vi "G heatmap=f(orbital angle, E_mol)_on Bi.vi"() -> ()   [LabVIEW 2016]
uses:
  <vilib>/Math Plots/3D Math Plots/3D Contour/3D Contour XCtrl/3D Contour.xctl
  <vilib>/Math Plots/3D Math Plots/3D Contour/3D Contour Datatype/3D Contour Datatype.lvclass
  <vilib>/Analysis/1siggen.llb/Ramp Pattern by Samples.vi
  <vilib>/Math Plots/3D Math Plots/3D Contour/3D Contour Datatype/Public/Plot Helper (Vector).vi
  <vilib>/Utility/file.llb/Write Delimited Spreadsheet (DBL).vi
  <vilib>/Analysis/NI_AALBase.lvlib
  <vilib>/Math Plots/3D Math Plots/3D Plot/3D Plot Datatype/3D Plot Datatype.lvclass
  <vilib>/Analysis/NI_AALPro.lvlib
panel:
  out "Array 3":dbl[](array[numeric])
  out "Array 2":dbl[](array[numeric])
  in  "turn on dyz":bool
  in  "turn on dz2":bool=TRUE
  out "<= min[dnn]?":bool
  out "e_FMO after dz2\n(vs. E_F) <=>\nintercept on E\ndz2 band-mol":dbl
  out "e_FMO after sp \n(vs. E_F) <=>\nintercept on E\nsp band-mol":dbl
  out "intercept on E\ndyz band-mol":dbl
  out "graphical sol_dyz band-mol":cluster{"Ramp Pattern":dbl[], dbl[]}[](graph)
  out "delta shift by d band \n(w.r.t. e_FMO coupled to s/p then dz2 )":dbl
  out "unweighted dyz SDOS \n@intercept":dbl
  in  "e_dyz band \n(vs. E_F)":dbl=-3.41 format="%.2f"
  in  "t_dyz band":dbl=1.1 format="%.2f"
  out "dyz SDOS top \n(/eV/atom)":dbl=0.793 format="%.3f"
  out "log(G/G0)=f(angle, e_iso) for t(sp-head)":refnum<class "3D Plot Datatype.lvclass">[](xcontrol)
  in  "min dnn (A)\nby induction":dbl=2.1 format="%.3g"
  out "Array":dbl[](array[numeric])
  out "peak value":dbl
  out "unweighted sp(xy) SDOS \n@ intercept":dbl
  out "t^2_sp(xy)-mol":dbl
  out "s/p(xy) SDOS top (/eV/atom)":dbl=0.118 format="%.3f"
  in  "e_s/p(xy) band (vs. E_F)":dbl=0.15 format="%.2f"
  in  "t_s/p(xy) band":dbl=2.99 format="%.2f"
  out "angle > ini?":bool
  in  "dnn shrinking \nrate\n(A/increment)":dbl=0.029 format="%.4g"
  in  "induction rate\n(_-fold of increment)":dbl=3.42 format="%.3g"
  in  "orbital angle \nstarting induction":dbl=47.14 format="%.2g"
  out "unweighted dz2 SDOS \n@intercept":dbl
  out "unweighted sp(z) SDOS \n@ intercept":dbl
  out "dz2 SDOS top \n(/eV/atom)":dbl=0.793 format="%.3f"
  out "s/p(z) SDOS top (/eV/atom)":dbl=0.118 format="%.3f"
  in  "eta scaling for sp":dbl=0.417 format="%.3f"
  in  "name (d band)":string="on Bi 6dz2"
  in  "saving path_heatmap (d band)":path=path "C:/Users/NTU/Desktop/project_BiUPD & PbUPD/modelling/general map on BiUPD"
  in  "save heatmap \n(d band)?":bool
  out "final ELA(angle, e_iso  for t(sp-head))":refnum<class "3D Plot Datatype.lvclass">[](xcontrol)
  out "delta(angle, e_iso) for t(d-head)_sum dz2 & dyz":refnum<class "3D Plot Datatype.lvclass">[](xcontrol)
  out "delta(angle, e_iso) for t(sp-head)_only pz":refnum<class "3D Plot Datatype.lvclass">[](xcontrol)
  out "delta shift by dz2 band \n(w.r.t. e_FMO coupled to s/p )":dbl
  out "delta shift by \nsp band":dbl
  in  "dnn (pi) dyz":dbl=100.0 format="%0.2f"
  out "Gamma(angle, e_iso) for t(sp-head)_sum pz & py":refnum<class "3D Plot Datatype.lvclass">[](xcontrol)
  out "e_FMO (vs. E_F)":dbl
  out "log(G/G0) matrix":dbl[][](array[numeric])
  in  "tilt (mol axis - Z axis)":dbl format="%0.2f"
  out "final ELA(angle, e_iso)  for t(d-head)":refnum<class "3D Plot Datatype.lvclass">[](xcontrol)
  out "Gamma(angle, e_iso) for t(d-head)_sum dz2 & dyz":refnum<class "3D Plot Datatype.lvclass">[](xcontrol)
  out "log(G/G0)=f(angle, e_iso) for t(d-head)":refnum<class "3D Plot Datatype.lvclass">[](xcontrol)
  out "e_FMO (y)":dbl[](array[numeric])
  out "angle\narray\nfor sigma":dbl[](array[numeric])
  in  "create heatmap":bool=TRUE
  in  "name (sp band)":string="on Bi 6pz 6pxy"
  in  "save heatmap \n(sp band)?":bool
  in  "saving path_heatmap (sp band)":path=path "C:/Users/NTU/Desktop/project_BiUPD & PbUPD/modelling/general map on BiUPD"
  in  "lower angle":dbl=-90.0 format="%_3g"
  in  "upper angle":dbl=90.0 format="%_3g"
  in  "angle increment":dbl=0.5 format="%_3g"
  in  "lower e_iso FMO":dbl=-3.0 format="%_3g"
  in  "upper e_iso FMO":dbl=3.0 format="%_3g"
  in  "increment_iso FMO":dbl=0.03 format="%_3g"
  out "t^2_dz2-mol":dbl
  out "FWHM (eV)":dbl
  in  "dnn (pi) p(xy)":dbl=2.61 format="%0.2f"
  in  "WF (eV) vs. Fermi":dbl format="%.2f"
  out "t^2_sp(z)-mol":dbl
  out "t_s/p(xy)-mol":dbl
  in  "eta (pi)":i32=3
  in  "start (eV)":dbl=-20.0 format="%.2f"
  in  "dnn (sigma) sp(z)":dbl=2.61 format="%0.2f"
  in  "eta (sigma)":i32=2
  out "t_sp(z)-mol":dbl
  out "intercept on E\nsp band-mol":dbl
  out "graphical sol_sp band-mol":cluster{"Ramp Pattern":dbl[], dbl[]}[](graph)
  in  "e_s/p(z) band (vs. E_F)":dbl=-0.6 format="%.2f"
  in  "t_s/p(z) band":dbl=2.71 format="%.2f"
  out "E":dbl[](array[numeric])
  out "t^2_dyz-mol":dbl
  out "final ELA (eV), via \n(1) sp intercept\n(2) dz2 intercept\n(3) dyz intercept":dbl
  in  "ELD AO (pi w/ FMO) - Z axis":dbl format="%0.2f"
  out "graphical sol_dz2 band-mol":cluster{"Ramp Pattern":dbl[], dbl[]}[](graph)
  out "intercept on E\ndz2 band-mol":dbl
  out "t_dz2-mol":dbl
  out "t_dyz-mol":dbl
  in  "e_dz2 band \n(vs. E_F)":dbl=14.41 format="%.2f"
  in  "t_dz2 band":dbl=5.1 format="%.2f"
  in  "eta (pi)":i32=2
  in  "ELD AO (sigma w/ FMO) - Z axis":dbl format="%0.2f"
  in  "mol backbone (# n)":dbl=8.0 format="%.2f"
  in  "beta (per n)":dbl=1.0 format="%.2f"
  out "conductance G0 \n(on E_F, low bias)":dbl format="%#.3e"
  in  "eta (sigma)":i32=1
  out "transmission T(E)":cluster{"Ramp Pattern":dbl[], dbl[]}(graph)
  in  "d state R (Ang)":dbl=1.0099999999999998 format="%0.2f"
  in  "FMO - mol axis":dbl format="%0.2f"
  in  "dnn (sigma) dz2":dbl=2.61 format="%0.2f"
  in  "samples":i32=10000
  in  "end (eV)":dbl=20.0 format="%_3g"
  # "for eld-head hopping integral: \nHarrsion and S-K"
  # "for ELA & Gamma: Hilbert & Newns-Anderson-Grimley graphical method"
  # "for T(E) and G(E_F)\nLandauer formula"
  # "logG heatmap = f(t(number basis), e_iso FMO)"
  # "step2. dz2 band-mol \ncoupling"
  # "step3. dyz band-mol coupling"
  # "step1. s/p band-mol coupling"
  # "Harrison LCAO hopping integral (V)"
  # "exp decay for backbone"
  # "internuclear \nspacing, dnn (Ang)"
  # "off-diagonal\nelement type"
  # "FMO-s/p eld AO"
  # "1 sp_sigma\n2 pp_sigma"
  # "1 sp_pi =0\n2 pp_sigma\n3 pp_pi"
  # "FMO-d eld AO"
  # "1 pd_sigma\n2 pd_pi"
  # "BiUPD dz2\nc: 14.41\nt: 5.10"
  # "the avg of the two \nshould be e_ELD (vs. E_F)"
  # "BiUPD dz2\nc: 14.41\nt: 5.10"
  # "Au dyz\nc: -3.41\nt: 1.10"
  # "Au s\nc: -0.04\nt: 5.03"
  # "Au py\nc: 11.01\nt: 6.11"
  # "BiUPD pz\nc: -0.60\nt: 2.71"
  # "BiUPD py\nc: 0.15\nt: 2.99"
  # "1 pd_sigma\n2 pd_pi"
  # "to switch off certain interactions => set very large d (Ang)"
  # "for heatmap"
  # "for inducting effect"
  # "e_iso FMO\n (vs. E_F)"
  # "angle basis"
  # "induction"
  # "dnn"
  # "note: this is\nnot simply \nthe Gamma"
  # "to switch off certain effects => set 1 or 0"
  # "Slater-Koster t =f(bond angle)"
  # "+"
  # "一"
  # "FMO - ELD AO \nangle (sigma)"
  # "="
  # "FMO - ELD AO\n angle (pi)"
  # "="
  # "inverse \ncolor scale"
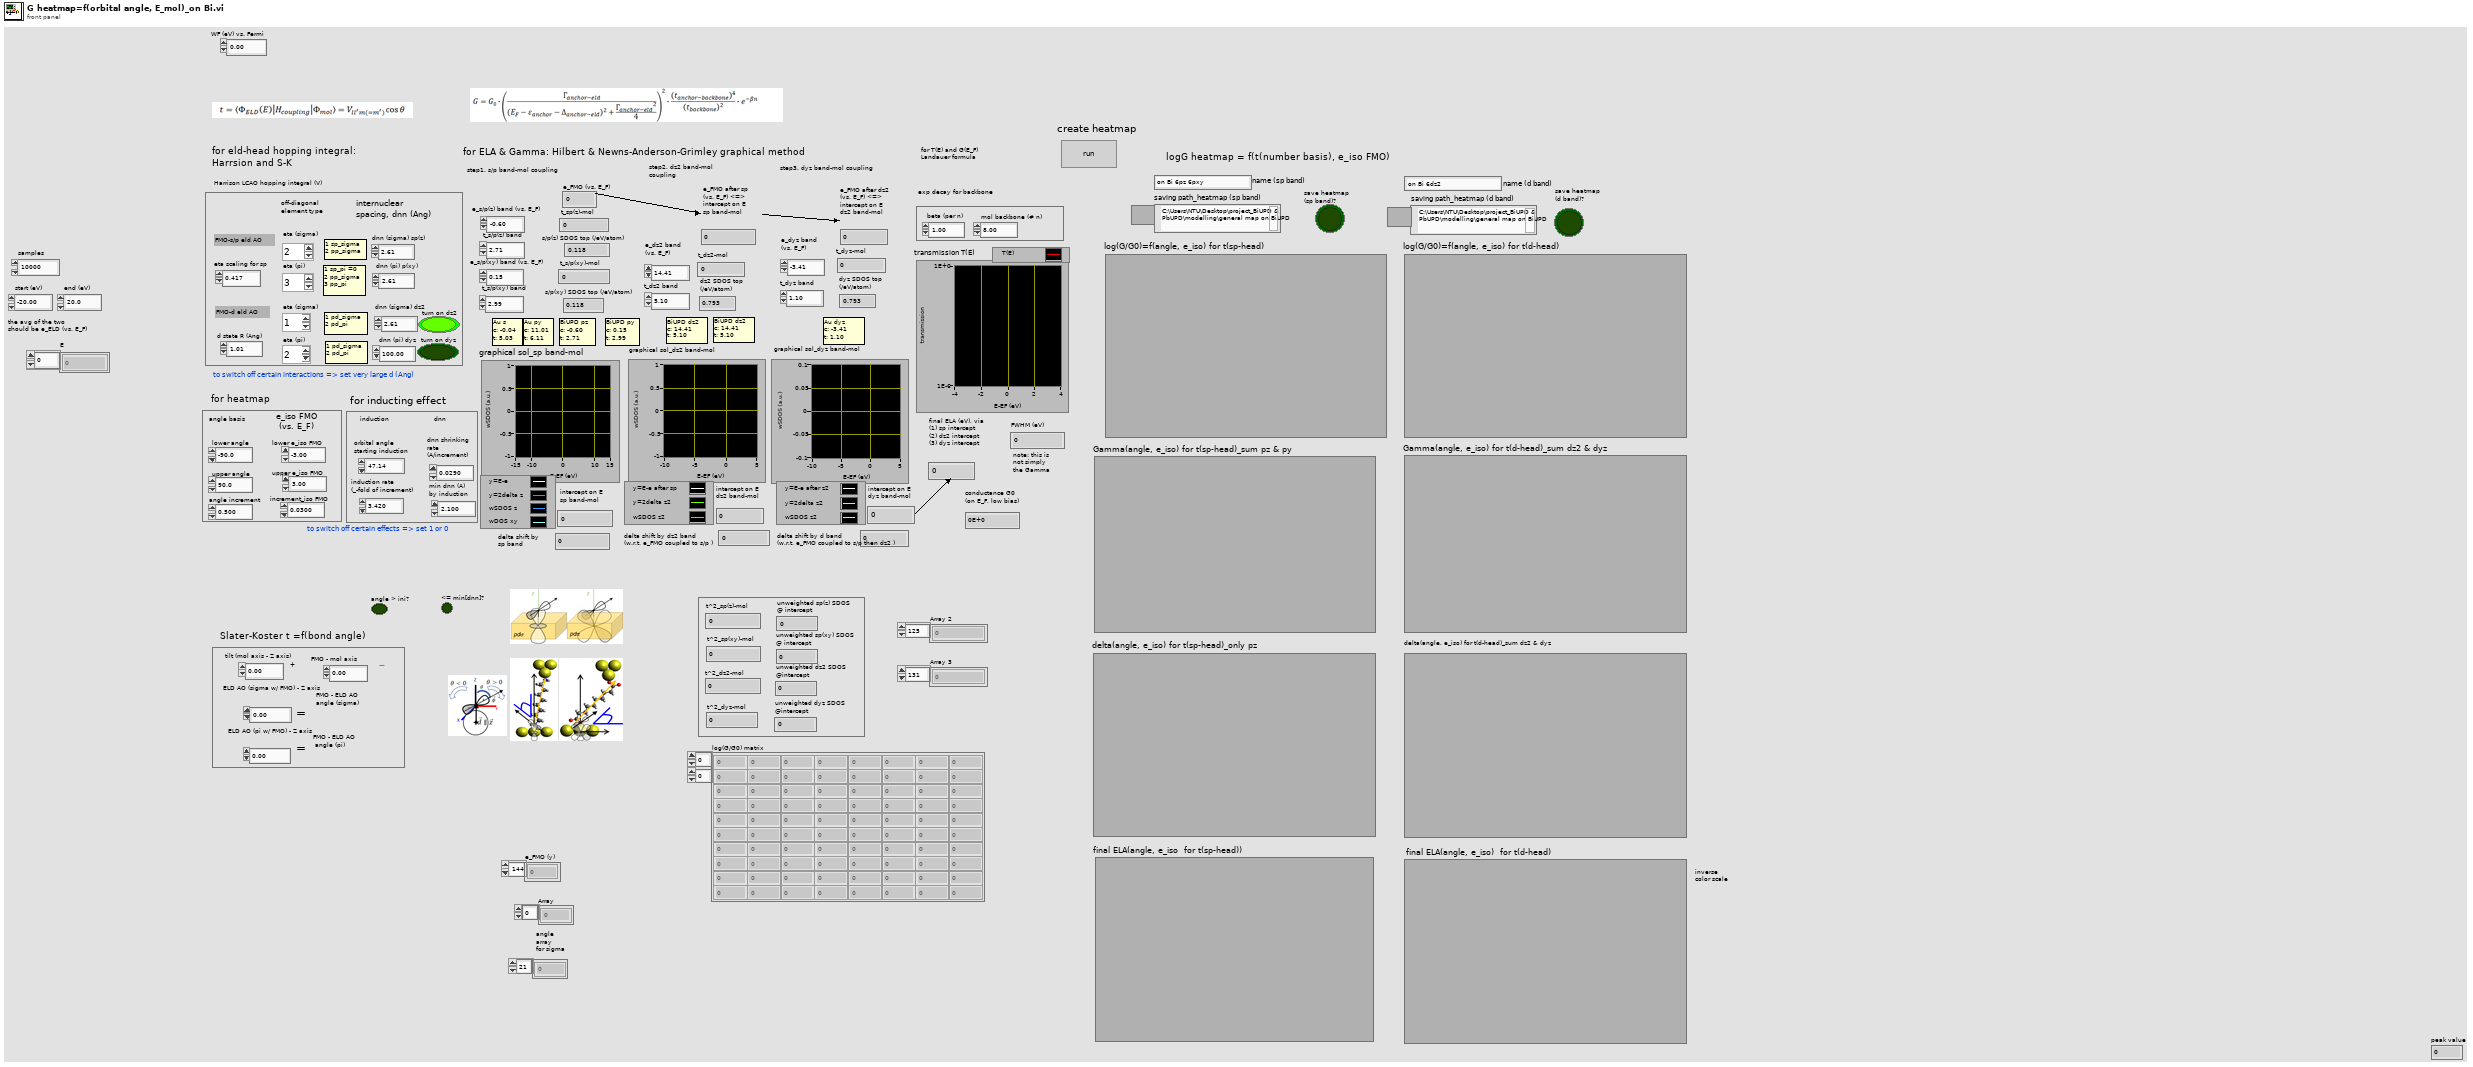
[diagram p1: front panel]
types:
  T1 = cluster{"Ramp Pattern":dbl[], "Hilbert{X}":dbl[]}
  T2 = cluster{"Ramp Pattern":dbl[], "Hilbert{X}":dbl[]}[]
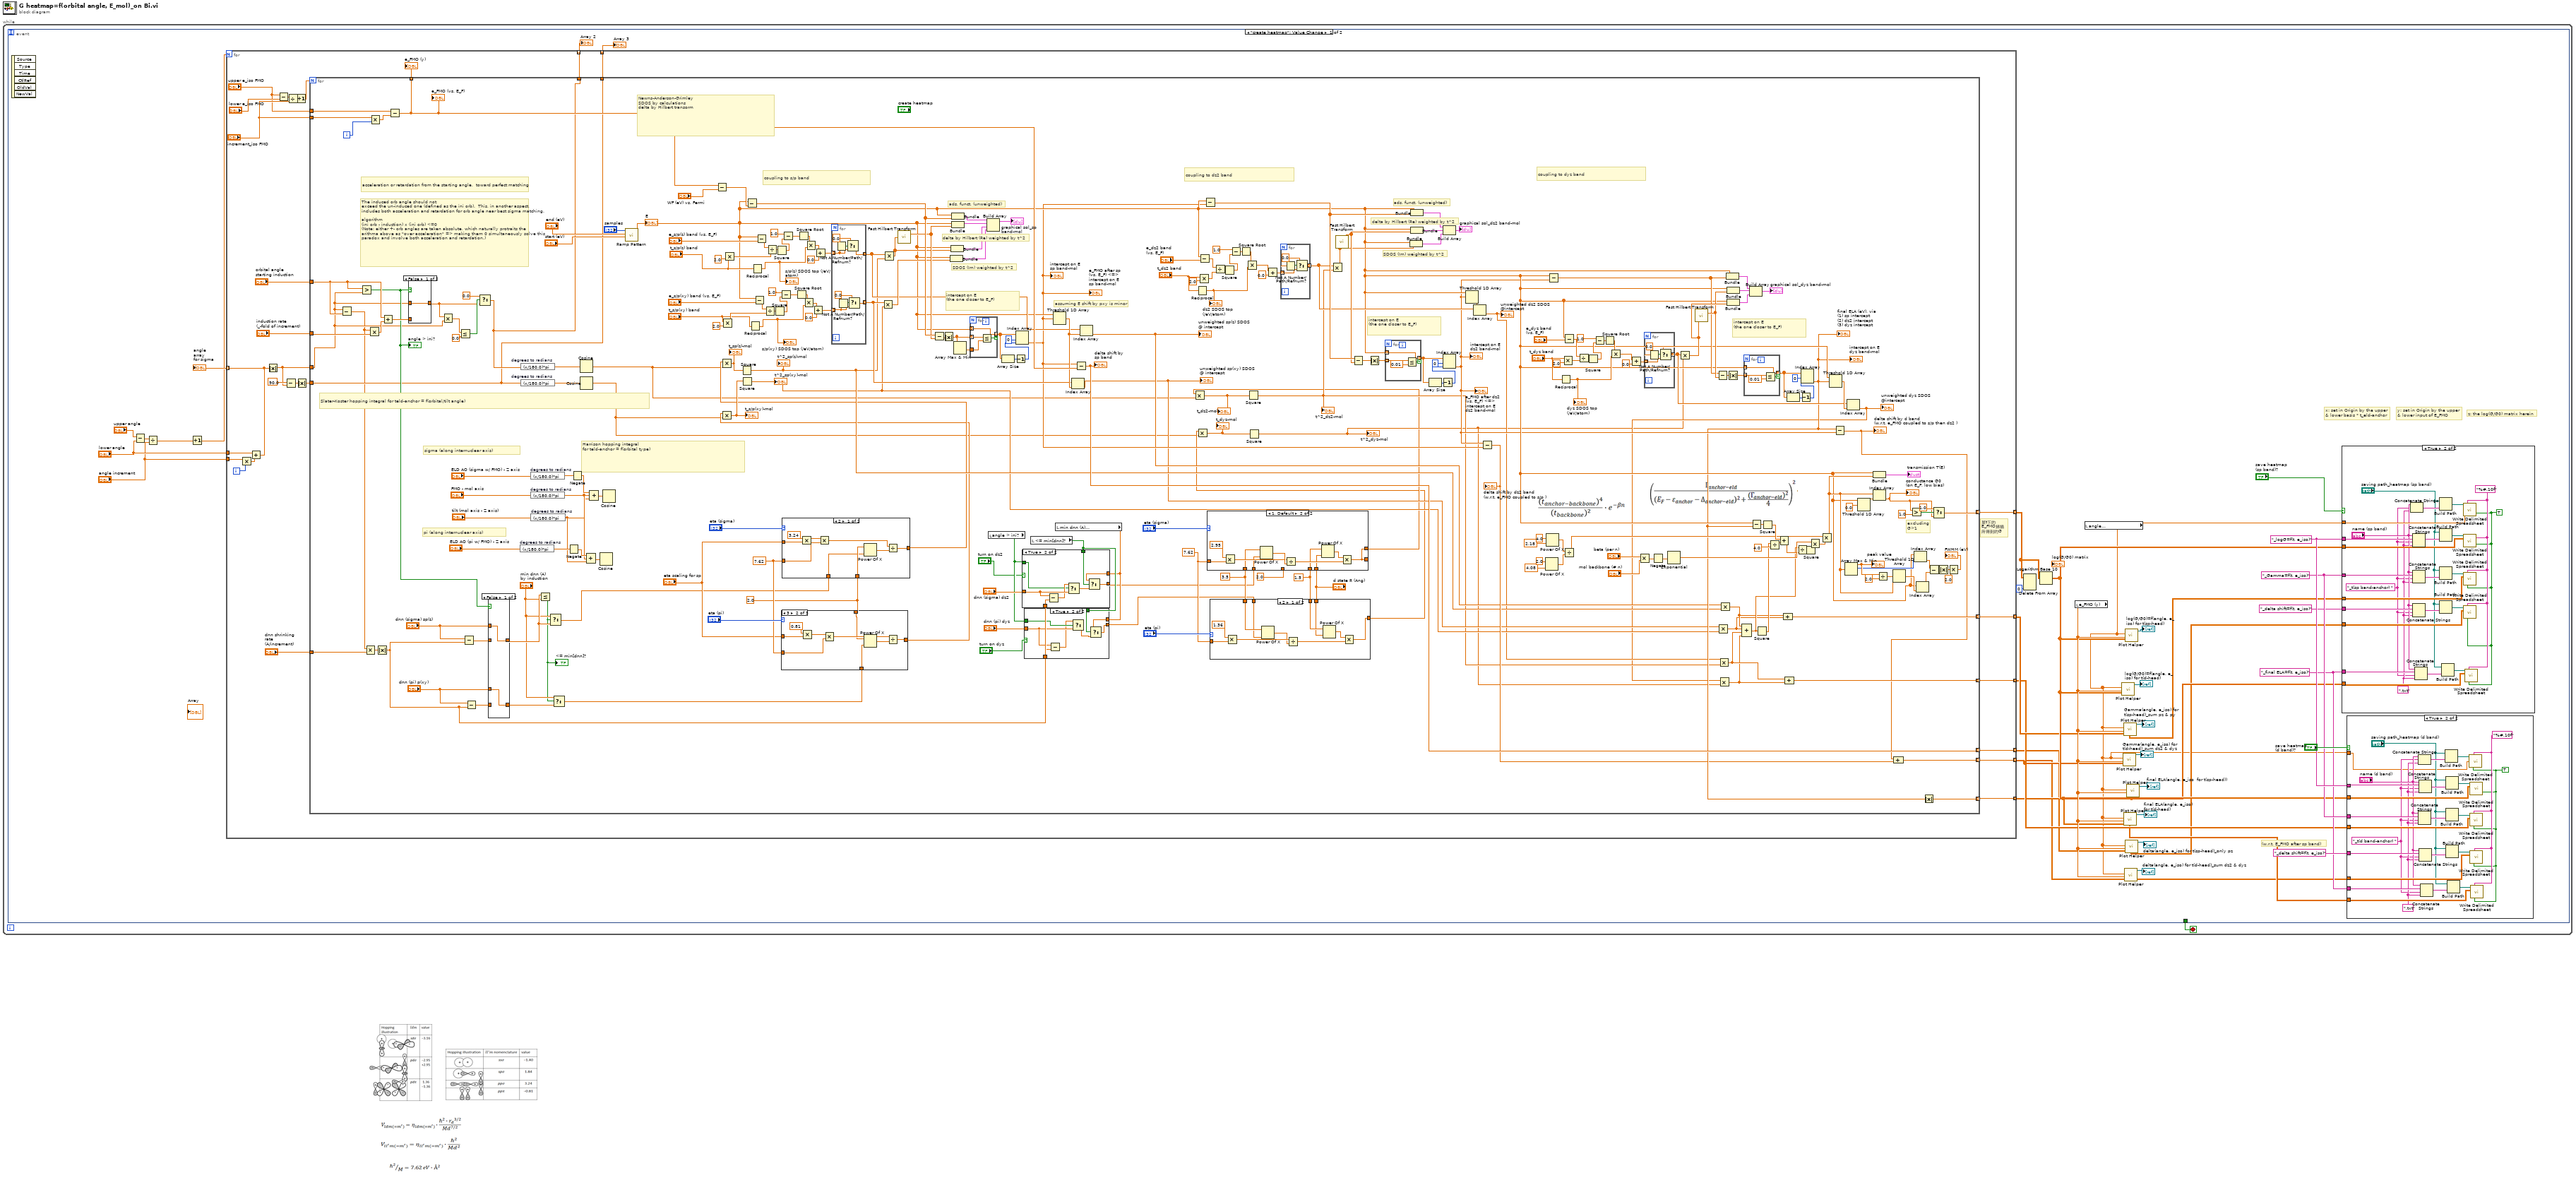
[diagram p0: block diagram]
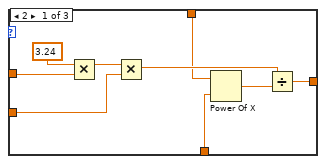
[diagram p8: hidden frame]
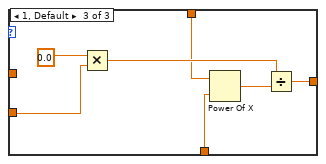
[diagram p9: hidden frame]
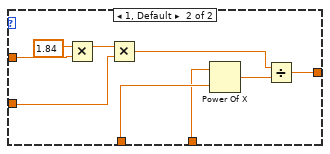
[diagram p10: hidden frame]
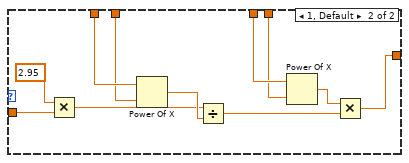
[diagram p11: hidden frame]
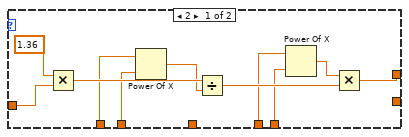
[diagram p12: hidden frame]
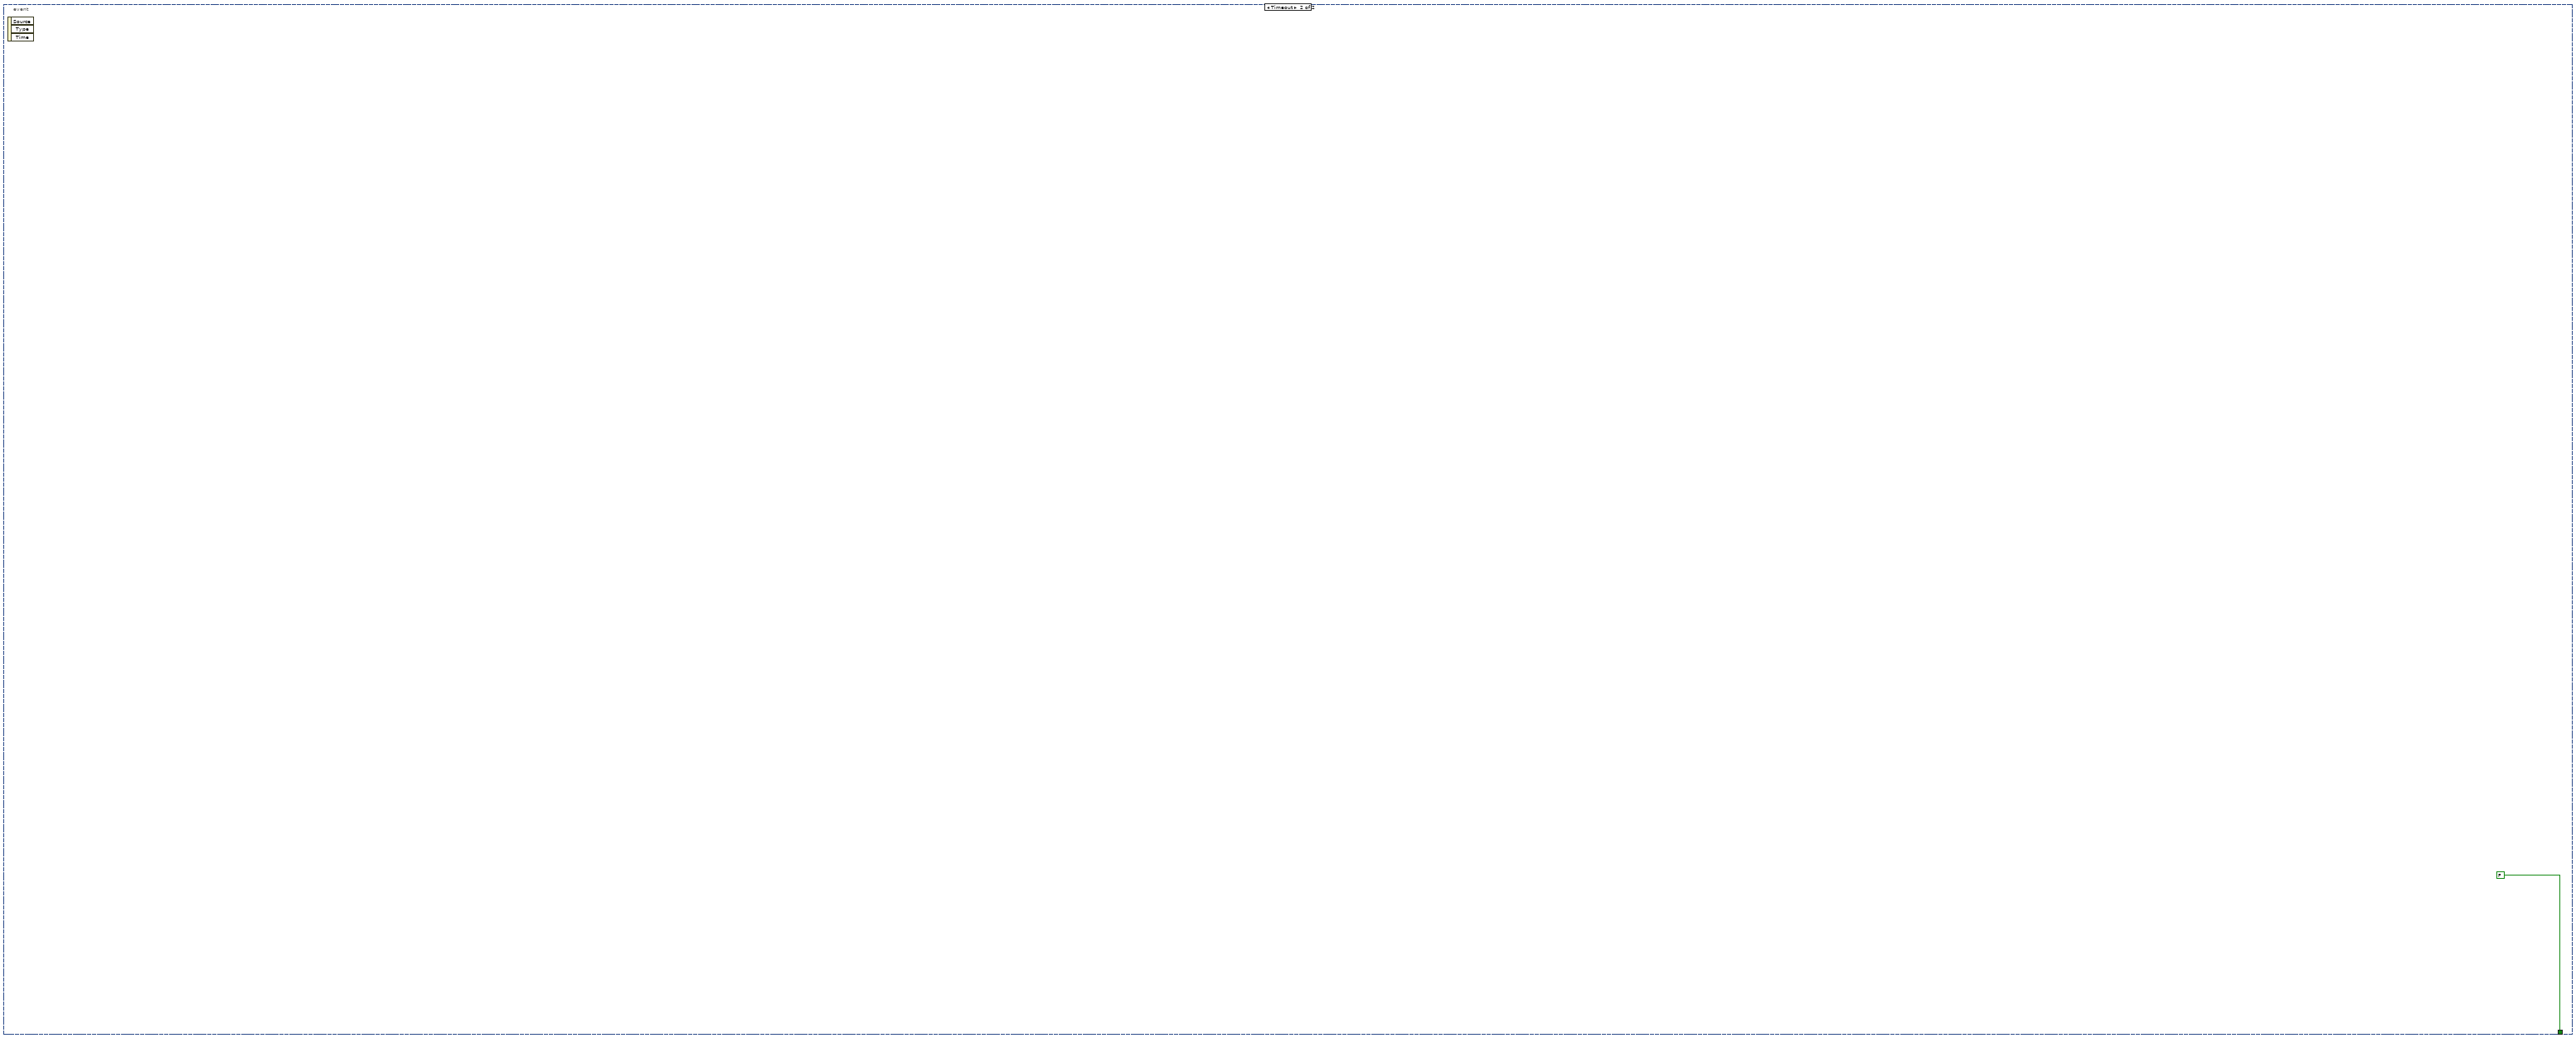
[diagram p13: hidden frame]
diagram:
  n1 = while {
    stop <- w1 stop-if-true
    n2 = event shown="[0] \"create heatmap\": Value Change" {
      selector: _ -> [_ _]
      dyn-events: _ -> [_ _]
      timeout: _ -> [_ _]
      tunnel: [_ FALSE] -> w1
      event "create heatmap": Value Change {
        w18 = "_logG=f(t, e_iso)" ("string")
        w14 = "_final ELA=f(t, e_iso)" ("string")
        w17 = "_Gamma=f(t, e_iso)" ("string")
        # "(w.r.t. E_FMO after sp band)"
        # "z: the log(G/G0) matrix herein"
        # "y: set in Origin by the upper \n& lower input of E_FMO"
        # "x: set in Origin by the upper\n& lower basis * t_eld-anchor"
        n3 = event-data() -> ()  [unwired: 1 in, 6 out]
        n4 = Subtract(x="upper angle", y="lower angle") -> (x-y=w34:dbl)
        n5 = Divide(x=w34, y="angle increment") -> (x/y=w35:dbl)
        n6 = Increment(x=w35) -> (x+1=w27:dbl)
        n7 = for {
          N: w27 -> [_]
          tunnel: "lower angle" -> [w102]
          tunnel: "angle increment" -> [w107]
          tunnel: [w97] -> w5 mode=indexing
          tunnel: [w92] -> w31 mode=indexing
          tunnel: [w105] -> w11 mode=indexing
          tunnel: [w104] -> w10 mode=indexing
          tunnel: [w100] -> w12 mode=indexing
          tunnel: [w99] -> w9 mode=indexing
          tunnel: [w98] -> w8 mode=indexing
          tunnel: [w87] -> w3 mode=indexing
          tunnel: [w86] -> w2 mode=indexing
          i -> [w108]
          # "某t下的\nE_FMO掃描\n所得到的G"
          n8 = Multiply(x=w107, y=w108) -> (x*y=w101:dbl)
          n9 = Add(x=w102, y=w101) -> (x+y=w92:dbl)
          n10 = Absolute Value(x=w92) -> (abs(x)=w90:dbl)
          n11 = Subtract(x="upper e_iso FMO", y="lower e_iso FMO") -> (x-y=w111:dbl)
          n12 = Subtract(x=90.0 ("y"), y=w90) -> (x-y=w91:dbl)
          n13 = Divide(x=w111, y="increment_iso FMO") -> (x/y=w112:dbl)
          n14 = Increment(x=w112) -> (x+1=w103:dbl)
          n15 = Absolute Value(x=w91) -> (abs(x)=w89:dbl)
          n16 = for {
            N: w103 -> [_]
            tunnel: "upper e_iso FMO" -> [w308]
            tunnel: "increment_iso FMO" -> [w307]
            tunnel: [w298] -> w106 mode=indexing
            tunnel: [w145] -> w105 mode=indexing
            tunnel: [w283] -> w104 mode=indexing
            tunnel: w90 -> [w195]
            tunnel: [w148] -> w100 mode=indexing
            tunnel: [w299] -> w99 mode=indexing
            tunnel: [w142] -> w98 mode=indexing
            tunnel: [w201] -> w97 mode=indexing
            tunnel: "orbital angle \nstarting induction" -> [w245]
            tunnel: "induction rate\n(_-fold of increment)" -> [w244]
            tunnel: "dnn shrinking \nrate\n(A/increment)" -> [w242]
            tunnel: w89 -> [w114]
            tunnel: [w114] -> w87
            tunnel: [w115] -> w86
            i -> [w309]
            w317 = 7.62
            w316 = 2.0
            w330 = 1.5
            w332 = 3.5
            w331 = 7.62
            # "acceleration or retardation from the starting angle,  toward perfect matching"
            # "intercept on E \n(the one closer to E_F)"
            # "coupling to dyz band"
            # "The induced orb angle should not \nexceed the un-induced one (defined as the ini orb).  This, in another aspect, includes both acceleration and retardation for orb angle near best sigma matching.\n\nalgorithm\n(ini orb - induction) x (ini orb) <=0\n(Note: either +- orb angles are taken absolute, which naturally protraits the arithma above as \"over acceleration\" => making them 0 simultaneously solve this paradox and involve both acceleration and retardation.)"
            # "assuming E shift by pxy is minor"
            # "excluding\nG>1"
            # "SDOS (Im) weighted by t^2"
            # "delta by Hilbert (Re) weighted by t^2"
            # "ads. funct. (unweighted)"
            # "SDOS (Im) weighted by t^2"
            # "delta by Hilbert (Re) weighted by t^2"
            # "ads. funct. (unweighted)"
            # "Newns-Anderson-Grimley \nSDOS by calculations\ndelta by Hilbert transorm"
            # "intercept on E \n(the one closer to E_F)"
            # "intercept on E \n(the one closer to E_F)"
            # "coupling to dz2 band"
            # "coupling to s/p band"
            # "Harrison hopping integral \nfor teld-anchor = f(orbital type)"
            # "pi (along internuclear axis)"
            # "sigma (along internuclear axis)"
            # "Slater-Koster hopping integral for teld-anchor = f(orbital/tilt angle)"
            n17 = Subtract(x=w195, y=w245) -> (x-y=w113:dbl)
            n18 = Greater?(x=w245, y=w195) -> (0:w239:bool)
            "angle > ini?" <- w239
            n19 = Multiply(x=w113, y=w242) -> (x*y=w243:dbl)
            n20 = Multiply(x=w113, y=w244) -> (x*y=w247:dbl)
            n21 = Multiply(x=w307, y=w309) -> (x*y=w310:dbl)
            n22 = Absolute Value(x=w243) -> (abs(x)=w236:dbl)
            n23 = Add(x=w245, y=w247) -> (x+y=w246:dbl)
            n24 = Subtract(x=w308, y=w310) -> (x-y=w298:dbl)
            "e_FMO (vs. E_F)" <- w298
            n25 = case shown="False" w239 {
              tunnel: w195 -> [w395 _]
              tunnel: [w395 w396] -> w196
              tunnel: w246 -> [_ w396]
              frame False {
              }
              frame True {
              }
            }
            n26 = Multiply(x=w196, y=w195) -> (x*y=w199:dbl)
            n27 = Less Or Equal?(x=w199, y=0.0) -> (x <= y?=w197:bool)
            n28 = Subtract(x="dnn (sigma) sp(z)", y=w236) -> (x-y=w241:dbl)
            n29 = Subtract(x="dnn (pi) p(xy)", y=w236) -> (x-y=w240:dbl)
            n30 = Select(t=0.0 ("y"), s=w197, f=w196) -> (s? t:f=w115:dbl)
            n31 = case shown="False" w239 {
              tunnel: w241 -> [_ w394]
              tunnel: [w392 w394] -> w194
              tunnel: w240 -> [_ w393]
              tunnel: [w391 w393] -> w193
              tunnel: "dnn (sigma) sp(z)" -> [w392 _]
              tunnel: "dnn (pi) p(xy)" -> [w391 _]
              frame False {
              }
              frame True {
              }
            }
            n32 = expression code="(x/180.0)*pi" "degrees to radians"("ELD AO (pi w/ FMO) - Z axis") -> (w347:dbl)
            n33 = expression code="(x/180.0)*pi" "degrees to radians"(w115) -> (w117:dbl)
            n34 = expression code="(x/180.0)*pi" "degrees to radians"(w114) -> (w116:dbl)
            n35 = expression code="(x/180.0)*pi" "degrees to radians"("ELD AO (sigma w/ FMO) - Z axis") -> (w351:dbl)
            n36 = expression code="(x/180.0)*pi" "degrees to radians"("FMO - mol axis") -> (w345:dbl)
            n37 = expression code="(x/180.0)*pi" "degrees to radians"("tilt (mol axis - Z axis)") -> (w311:dbl)
            n38 = Less Or Equal?(x=w194, y="min dnn (A)\nby induction") -> (x <= y?=w191:bool)
            "<= min[dnn]?" <- w191
            n39 = Select(t="min dnn (A)\nby induction", s=w191, f=w194) -> (s? t:f=w124:dbl)
            n40 = Select(t="min dnn (A)\nby induction", s=w191, f=w193) -> (s? t:f=w190:dbl)
            n41 = Negate(x=w347) -> (-x=w346:dbl)
            n42 = Negate(x=w351) -> (-x=w348:dbl)
            n43 = Cosine(x=w117) -> (cos(x)=w118:dbl)
            n44 = Cosine(x=w116) -> (cos(x)=w119:dbl)
            n45 = Compound Arithmetic op=ADD(w346, w345, w311) -> (w349:dbl)
            n46 = Compound Arithmetic op=ADD(w348, w345, w311) -> (w354:dbl)
            n47 = Cosine(x=w349) -> ()  [unwired: 1 out]
            n48 = Cosine(x=w354) -> ()  [unwired: 1 out]
            n49 = call-poly <vilib>:"Ramp Pattern.vi"("start"="start (eV)", "end"="end (eV)", "samples"="samples") -> ("Ramp Pattern"=w154:dbl[])  [unwired: 7 in, 1 out]
            "E" <- w154
            n50 = Subtract(x=w298, y="WF (eV) vs. Fermi") -> (x-y=w312:dbl)
            n51 = Multiply(x="t_s/p(xy) band", y=2.0) -> (x*y=w233:dbl)
            n52 = Multiply(x="t_s/p(z) band", y=2.0) -> (x*y=w235:dbl)
            n53 = Subtract(x=w154, y=w312) -> (x-y=w355:dbl[])
            n54 = Reciprocal(x="t_s/p(xy) band") -> (1/x=w223:dbl)
            "s/p(xy) SDOS top (/eV/atom)" <- w223
            n55 = Reciprocal(x="t_s/p(z) band") -> (1/x=w234:dbl)
            "s/p(z) SDOS top (/eV/atom)" <- w234
            n56 = Subtract(x=w154, y="e_s/p(xy) band (vs. E_F)") -> (x-y=w225:dbl[])
            n57 = Subtract(x=w154, y="e_s/p(z) band (vs. E_F)") -> (x-y=w280:dbl[])
            n58 = Divide(x=w225, y=w233) -> (x/y=w227:dbl[])
            n59 = Divide(x=w280, y=w235) -> (x/y=w278:dbl[])
            n60 = Square(x=w227) -> (x^2=w228:dbl[])
            n61 = Square(x=w278) -> (x^2=w277:dbl[])
            n62 = Subtract(x=1.0, y=w228) -> (x-y=w229:dbl[])
            n63 = case shown="3" "eta (pi)" {
              tunnel: w317 -> [w413 w423 w430]
              tunnel: [w412 w422 w429] -> w122
              tunnel: w316 -> [w414 w421 w428]
              tunnel: w190 -> [w411 w420 w427]
              tunnel: "eta scaling for sp" -> [w409 w418 _]
              frame 2 {
                n64 = Multiply(x=3.24, y=w409) -> (x*y=w410:dbl)
                n65 = Multiply(x=w410, y=w413) -> (x*y=w416:dbl)
                n66 = Power Of X(1:w411, 2:w414) -> (0:w415:dbl)
                n67 = Divide(x=w416, y=w415) -> (x/y=w412:dbl)
              }
              frame 3 {
                n68 = Multiply(x=0.81, y=w418) -> (x*y=w419:dbl)
                n69 = Multiply(x=w419, y=w423) -> (x*y=w425:dbl)
                n70 = Power Of X(1:w420, 2:w421) -> (0:w426:dbl)
                n71 = Divide(x=w425, y=w426) -> (x/y=w422:dbl)
              }
              frame 1, Default {
                n72 = Multiply(x=0.0, y=w430) -> (x*y=w432:dbl)
                n73 = Power Of X(1:w427, 2:w428) -> (0:w433:dbl)
                n74 = Divide(x=w432, y=w433) -> (x/y=w429:dbl)
              }
            }
            n75 = Multiply(x=w122, y=w119) -> (x*y=w303:dbl)
            "t_s/p(xy)-mol" <- w303
            n76 = Square(x=w303) -> (x^2=w138:dbl)
            "t^2_sp(xy)-mol" <- w138
            n77 = Subtract(x=1.0, y=w277) -> (x-y=w276:dbl[])
            n78 = case shown="2" "eta (sigma)" {
              tunnel: w317 -> [w439 w450]
              tunnel: [w436 w447] -> w123
              tunnel: w124 -> [w437 w449]
              tunnel: w316 -> [w440 w448]
              tunnel: "eta scaling for sp" -> [w434 w443]
              frame 2 {
                n79 = Multiply(x=3.24, y=w434) -> (x*y=w435:dbl)
                n80 = Multiply(x=w435, y=w439) -> (x*y=w441:dbl)
                n81 = Power Of X(1:w437, 2:w440) -> (0:w442:dbl)
                n82 = Divide(x=w441, y=w442) -> (x/y=w436:dbl)
              }
              frame 1, Default {
                n83 = Multiply(x=1.84, y=w443) -> (x*y=w444:dbl)
                n84 = Multiply(x=w444, y=w450) -> (x*y=w446:dbl)
                n85 = Power Of X(1:w449, 2:w448) -> (0:w445:dbl)
                n86 = Divide(x=w446, y=w445) -> (x/y=w447:dbl)
              }
            }
            n87 = Multiply(x=w123, y=w118) -> (x*y=w302:dbl)
            "t_sp(z)-mol" <- w302
            n88 = Square(x=w302) -> (x^2=w140:dbl)
            "t^2_sp(z)-mol" <- w140
            n89 = Square Root(x=w229) -> (sqrt(x)=w230:dbl[])
            n90 = Square Root(x=w276) -> (sqrt(x)=w275:dbl[])
            n91 = Multiply(x=w230, y=w223) -> (x*y=w231:dbl[])
            n92 = Multiply(x=w275, y=w234) -> (x*y=w274:dbl[])
            n93 = Add(x=w231, y=0.0) -> (x+y=w221:dbl[])
            n94 = Add(x=w274, y=0.0) -> (x+y=w272:dbl[])
            n95 = for {
              tunnel: w272 -> [w405] mode=indexing
              tunnel: [w407] -> w188 mode=indexing
              tunnel: w221 -> [w402] mode=indexing
              tunnel: [w401] -> w189 mode=indexing
              n96 = Not A Number/Path/Refnum?(number/path/refnum=w405) -> (NaN/Path/Refnum?=w408:bool)
              n97 = Not A Number/Path/Refnum?(number/path/refnum=w402) -> (NaN/Path/Refnum?=w403:bool)
              n98 = Select(t=0.0, s=w408, f=w405) -> (s? t:f=w407:dbl)
              n99 = Select(t=0.0, s=w403, f=w402) -> (s? t:f=w401:dbl)
            }
            n100 = Multiply(x=w189, y=w138) -> (x*y=w205:dbl[])
            n101 = Multiply(x=w188, y=w140) -> (x*y=w266:dbl[])
            n102 = call <vilib>:"Fast Hilbert Transform.vi"("X"=w266) -> ("Hilbert{X}"=w269:dbl[])  [unwired: 1 out]
            n103 = Subtract(x=w355, y=w269) -> (x-y=w324:dbl[])
            n104 = Absolute Value(x=w324) -> (abs(x)=w268:dbl[])
            n105 = Bundle("Ramp Pattern"=w154, w205) -> (w204:cluster{"Ramp Pattern":dbl[], dbl[]})  [unwired: 1 in]
            n106 = Bundle("Ramp Pattern"=w154, w266) -> (w270:cluster{"Ramp Pattern":dbl[], dbl[]})  [unwired: 1 in]
            n107 = Bundle("Ramp Pattern"=w154, "Hilbert{X}"=w269) -> (w325:T1)  [unwired: 1 in]
            n108 = Bundle("Ramp Pattern"=w154, w355) -> (w327:cluster{"Ramp Pattern":dbl[], dbl[]})  [unwired: 1 in]
            n109 = Array Max & Min(array=w268) -> (min value=w267:dbl)  [unwired: 3 out]
            n110 = for {
              tunnel: w268 -> [w455] mode=indexing
              tunnel: [w453] -> w323 mode=indexing if=w454
              tunnel: w154 -> [w453] mode=indexing
              tunnel: w267 -> [w452]
              n111 = Less Or Equal?(x=w455, y=w452) -> (x <= y?=w454:bool)
            }
            n112 = Build Array(w327, w325, w270, w204) -> (→"graphical sol_sp band-mol":T2)
            n113 = local read "angle > ini?"() -> (w132:bool)
            n114 = Array Size(array=w323) -> (size(s)=w321:i32)
            n115 = Decrement(x=w321) -> (x-1=w320:i32)
            n116 = Index Array(array=w323, index #1=0 ("index"), index #2=w320) -> (element #2=w153:dbl)  [unwired: 1 out]
            "intercept on E\nsp band-mol" <- w153
            "e_FMO after sp \n(vs. E_F) <=>\nintercept on E\nsp band-mol" <- w153
            n117 = local read "<= min[dnn]?"() -> (w128:bool)
            n118 = Threshold 1D Array(2:w153, 3:w154) -> (0:w220:dbl)  [unwired: 1 in]
            n119 = local read "min dnn (A)\nby induction"() -> (w127:dbl)
            n120 = case shown="True" "turn on dz2" {
              tunnel: w236 -> [_ w382]
              tunnel: "dnn (sigma) dz2" -> [w374 w381]
              tunnel: w132 -> [_ w379]
              tunnel: w128 -> [_ w378]
              tunnel: w127 -> [_ w377]
              tunnel: [w374 w375] -> w126
              frame False {
              }
              frame True {
                n121 = Subtract(x=w381, y=w382) -> (x-y=w380:dbl)
                n122 = Select(t=w380, s=w379, f=w381) -> (s? t:f=w376:dbl)
                n123 = Select(t=w377, s=w378, f=w376) -> (s? t:f=w375:dbl)
              }
            }
            n124 = case shown="True" "turn on dyz" {
              tunnel: w236 -> [_ w373]
              tunnel: w132 -> [_ w372]
              tunnel: "dnn (pi) dyz" -> [w365 w371]
              tunnel: [w365 w366] -> w125
              tunnel: w128 -> [_ w369]
              tunnel: w127 -> [_ w368]
              frame False {
              }
              frame True {
                n125 = Subtract(x=w371, y=w373) -> (x-y=w370:dbl)
                n126 = Select(t=w370, s=w372, f=w371) -> (s? t:f=w367:dbl)
                n127 = Select(t=w368, s=w369, f=w367) -> (s? t:f=w366:dbl)
              }
            }
            n128 = Index Array(array=w189, index=w220) -> (element=w139:dbl)
            "unweighted sp(xy) SDOS \n@ intercept" <- w139
            n129 = Subtract(x=w153, y=w298) -> (x-y=w299:dbl)
            "delta shift by \nsp band" <- w299
            n130 = Index Array(array=w188, index=w220) -> (element=w141:dbl)
            "unweighted sp(z) SDOS \n@ intercept" <- w141
            n131 = Reciprocal(x="t_dz2 band") -> (1/x=w184:dbl)
            "dz2 SDOS top \n(/eV/atom)" <- w184
            n132 = Multiply(x="t_dz2 band", y=2.0) -> (x*y=w255:dbl)
            n133 = Subtract(x=w154, y="e_dz2 band \n(vs. E_F)") -> (x-y=w257:dbl[])
            n134 = Subtract(x=w154, y=w153) -> (x-y=w357:dbl[])
            n135 = case shown="1, Default" "eta (sigma)" {
              tunnel: w331 -> [w483 w499]
              tunnel: [w478 w489] -> w121
              tunnel: w126 -> [w481 w494]
              tunnel: w332 -> [w482 w493]
              tunnel: w330 -> [w480 w492]
              tunnel: "d state R (Ang)" -> [w479 w491]
              tunnel: 2.0 -> [_ _]
              tunnel: [_ w489] -> _
              frame 2 {
                n136 = Multiply(x=1.36, y=w483) -> (x*y=w485:dbl)
                n137 = Power Of X(1:w481, 2:w482) -> (0:w484:dbl)
                n138 = Divide(x=w485, y=w484) -> (x/y=w486:dbl)
                n139 = Power Of X(1:w479, 2:w480) -> (0:w487:dbl)
                n140 = Multiply(x=w487, y=w486) -> (x*y=w478:dbl)
              }
              frame 1, Default {
                n141 = Multiply(x=2.95, y=w499) -> (x*y=w497:dbl)
                n142 = Power Of X(1:w494, 2:w493) -> (0:w498:dbl)
                n143 = Divide(x=w497, y=w498) -> (x/y=w496:dbl)
                n144 = Power Of X(1:w491, 2:w492) -> (0:w495:dbl)
                n145 = Multiply(x=w495, y=w496) -> (x*y=w489:dbl)
              }
            }
            n146 = Multiply(x=w121, y=w118) -> (x*y=w305:dbl)
            "t_dz2-mol" <- w305
            n147 = case shown="2" "eta (pi)" {
              tunnel: w331 -> [w461 w477]
              tunnel: [w460 w472] -> w120
              tunnel: w332 -> [w459 w470]
              tunnel: w125 -> [w458 w469]
              tunnel: w330 -> [w457 w468]
              tunnel: "d state R (Ang)" -> [w456 w467]
              frame 2 {
                n148 = Multiply(x=1.36, y=w461) -> (x*y=w463:dbl)
                n149 = Power Of X(1:w458, 2:w459) -> (0:w462:dbl)
                n150 = Divide(x=w463, y=w462) -> (x/y=w464:dbl)
                n151 = Power Of X(1:w456, 2:w457) -> (0:w465:dbl)
                n152 = Multiply(x=w465, y=w464) -> (x*y=w460:dbl)
              }
              frame 1, Default {
                n153 = Multiply(x=2.95, y=w477) -> (x*y=w475:dbl)
                n154 = Power Of X(1:w469, 2:w470) -> (0:w476:dbl)
                n155 = Divide(x=w475, y=w476) -> (x/y=w474:dbl)
                n156 = Power Of X(1:w467, 2:w468) -> (0:w473:dbl)
                n157 = Multiply(x=w473, y=w474) -> (x*y=w472:dbl)
              }
            }
            n158 = Multiply(x=w120, y=w119) -> (x*y=w304:dbl)
            "t_dyz-mol" <- w304
            n159 = Divide(x=w257, y=w255) -> (x/y=w259:dbl[])
            n160 = Square(x=w259) -> (x^2=w260:dbl[])
            n161 = Subtract(x=1.0, y=w260) -> (x-y=w261:dbl[])
            n162 = Square Root(x=w261) -> (sqrt(x)=w262:dbl[])
            n163 = Multiply(x=w262, y=w184) -> (x*y=w263:dbl[])
            n164 = Square(x=w305) -> (x^2=w136:dbl)
            "t^2_dz2-mol" <- w136
            n165 = Square(x=w304) -> (x^2=w134:dbl)
            "t^2_dyz-mol" <- w134
            n166 = Add(x=w263, y=0.0) -> (x+y=w265:dbl[])
            n167 = for {
              tunnel: w265 -> [w397] mode=indexing
              tunnel: [w399] -> w187 mode=indexing
              n168 = Not A Number/Path/Refnum?(number/path/refnum=w397) -> (NaN/Path/Refnum?=w400:bool)
              n169 = Select(t=0.0, s=w400, f=w397) -> (s? t:f=w399:dbl)
            }
            n170 = Multiply(x=w187, y=w136) -> (x*y=w252:dbl[])
            n171 = call <vilib>:"Fast Hilbert Transform.vi"("X"=w252) -> ("Hilbert{X}"=w254:dbl[])  [unwired: 1 out]
            n172 = Subtract(x=w357, y=w254) -> (x-y=w340:dbl[])
            n173 = Absolute Value(x=w340) -> (abs(x)=w251:dbl[])
            n174 = for {
              tunnel: w251 -> [w503] mode=indexing
              tunnel: [w501] -> w339 mode=indexing if=w502
              tunnel: w154 -> [w501] mode=indexing
              n175 = Less Or Equal?(x=w503, y=0.01) -> (x <= y?=w502:bool)
            }
            n176 = Bundle("Ramp Pattern"=w154, w252) -> (w253:cluster{"Ramp Pattern":dbl[], dbl[]})  [unwired: 1 in]
            n177 = Bundle("Ramp Pattern"=w154, w357) -> (w343:cluster{"Ramp Pattern":dbl[], dbl[]})  [unwired: 1 in]
            n178 = Bundle("Ramp Pattern"=w154, "Hilbert{X}"=w254) -> (w341:T1)  [unwired: 1 in]
            n179 = Array Size(array=w339) -> (size(s)=w337:i32)
            n180 = Decrement(x=w337) -> (x-1=w336:i32)
            n181 = Index Array(array=w339, index #1=0 ("index"), index #2=w336) -> (element #2=w152:dbl)  [unwired: 1 out]
            "intercept on E\ndz2 band-mol" <- w152
            "e_FMO after dz2\n(vs. E_F) <=>\nintercept on E\ndz2 band-mol" <- w152
            n182 = Build Array(w343, w341, w253) -> (→"graphical sol_dz2 band-mol":T2)
            n183 = Threshold 1D Array(2:w152, 3:w154) -> (0:w186:dbl)  [unwired: 1 in]
            n184 = Index Array(array=w187, index=w186) -> (element=w137:dbl)
            "unweighted dz2 SDOS \n@intercept" <- w137
            n185 = Subtract(x=w152, y=w153) -> (x-y=w144:dbl)
            "delta shift by dz2 band \n(w.r.t. e_FMO coupled to s/p )" <- w144
            n186 = Power Of X(1:4.08, 2:2.0 ("x")) -> (0:w290:dbl)
            n187 = Power Of X(1:2.18, 2:4.0 ("x")) -> (0:w291:dbl)
            n188 = Subtract(x=w154, y=w152) -> (x-y=w161:dbl[])
            n189 = Reciprocal(x="t_dyz band") -> (1/x=w183:dbl)
            "dyz SDOS top \n(/eV/atom)" <- w183
            n190 = Multiply(x="t_dyz band", y=2.0) -> (x*y=w181:dbl)
            n191 = Subtract(x=w154, y="e_dyz band \n(vs. E_F)") -> (x-y=w179:dbl[])
            n192 = Divide(x=w291, y=w290) -> (x/y=w284:dbl)
            n193 = Divide(x=w179, y=w181) -> (x/y=w177:dbl[])
            n194 = Square(x=w177) -> (x^2=w176:dbl[])
            n195 = Subtract(x=1.0, y=w176) -> (x-y=w175:dbl[])
            n196 = Square Root(x=w175) -> (sqrt(x)=w174:dbl[])
            n197 = Multiply(x=w174, y=w183) -> (x*y=w173:dbl[])
            n198 = Add(x=w173, y=0.0) -> (x+y=w171:dbl[])
            n199 = Multiply(x="beta (per n)", y="mol backbone (# n)") -> (x*y=w301:dbl)
            n200 = for {
              tunnel: w171 -> [w387] mode=indexing
              tunnel: [w389] -> w159 mode=indexing
              n201 = Not A Number/Path/Refnum?(number/path/refnum=w387) -> (NaN/Path/Refnum?=w390:bool)
              n202 = Select(t=0.0, s=w390, f=w387) -> (s? t:f=w389:dbl)
            }
            n203 = Negate(x=w301) -> (-x=w358:dbl)
            n204 = Exponential(1:w358) -> (0:w300:dbl)
            n205 = Multiply(x=w159, y=w134) -> (x*y=w169:dbl[])
            n206 = call <vilib>:"Fast Hilbert Transform.vi"("X"=w169) -> ("Hilbert{X}"=w162:dbl[])  [unwired: 1 out]
            n207 = Subtract(x=w161, y=w162) -> (x-y=w163:dbl[])
            n208 = Multiply(x=w139, y=w138) -> (x*y=w149:dbl)
            n209 = Multiply(x=w137, y=w136) -> (x*y=w147:dbl)
            n210 = Multiply(x=w141, y=w140) -> (x*y=w150:dbl)
            n211 = Bundle("Ramp Pattern"=w154, w161) -> (w158:cluster{"Ramp Pattern":dbl[], dbl[]})  [unwired: 1 in]
            n212 = Bundle("Ramp Pattern"=w154, w169) -> (w156:cluster{"Ramp Pattern":dbl[], dbl[]})  [unwired: 1 in]
            n213 = Absolute Value(x=w163) -> (abs(x)=w168:dbl[])
            n214 = Bundle("Ramp Pattern"=w154, "Hilbert{X}"=w162) -> (w157:T1)  [unwired: 1 in]
            n215 = for {
              tunnel: w168 -> [w386] mode=indexing
              tunnel: [w384] -> w164 mode=indexing if=w385
              tunnel: w154 -> [w384] mode=indexing
              n216 = Less Or Equal?(x=w386, y=0.01) -> (x <= y?=w385:bool)
            }
            n217 = Build Array(w158, w157, w156) -> (→"graphical sol_dyz band-mol":T2)
            n218 = Compound Arithmetic op=ADD(w150, w149) -> (w148:dbl)
            n219 = Array Size(array=w164) -> (size(s)=w166:i32)
            n220 = Decrement(x=w166) -> (x-1=w167:i32)
            n221 = Index Array(array=w164, index #1=0 ("index"), index #2=w167) -> (element #2=w151:dbl)  [unwired: 1 out]
            "final ELA (eV), via \n(1) sp intercept\n(2) dz2 intercept\n(3) dyz intercept" <- w151
            "intercept on E\ndyz band-mol" <- w151
            n222 = Subtract(x=w154, y=w151) -> (x-y=w364:dbl[])
            n223 = Square(x=w364) -> (x^2=w296:dbl[])
            n224 = Threshold 1D Array(2:w151, 3:w154) -> (0:w160:dbl)  [unwired: 1 in]
            n225 = Subtract(x=w151, y=w152) -> (x-y=w143:dbl)
            "delta shift by d band \n(w.r.t. e_FMO coupled to s/p then dz2 )" <- w143
            n226 = Index Array(array=w159, index=w160) -> (element=w135:dbl)
            "unweighted dyz SDOS \n@intercept" <- w135
            n227 = Multiply(x=w135, y=w134) -> (x*y=w146:dbl)
            n228 = Compound Arithmetic op=ADD(w150, w149, w147, w146) -> (w203:dbl)
            n229 = Square(x=w203) -> (x^2=w286:dbl)
            n230 = Divide(x=w286, y=4.0 ("x")) -> (x/y=w294:dbl)
            n231 = Add(x=w296, y=w294) -> (x+y=w295:dbl[])
            n232 = Compound Arithmetic op=ADD(w147, w146) -> (w145:dbl)
            n233 = Divide(x=w203, y=w295) -> (x/y=w356:dbl[])
            n234 = Square(x=w356) -> (x^2=w285:dbl[])
            n235 = Multiply(x=w300, y=w285) -> (x*y=w297:dbl[])
            n236 = Multiply(x=w284, y=w297) -> (x*y=w207:dbl[])
            n237 = Array Max & Min(array=w207) -> (max value=w217:dbl, max index (indices)=w209:i32)  [unwired: 2 out]
            "peak value" <- w217
            n238 = Threshold 1D Array(2:0.0 ("threshold y"), 3:w154) -> (0:w361:dbl)  [unwired: 1 in]
            n239 = Index Array(array=w207, index=w361) -> (element=w202:dbl)
            "conductance G0 \n(on E_F, low bias)" <- w202
            n240 = Bundle("Ramp Pattern"=w154, w207) -> (→"transmission T(E)":cluster{"Ramp Pattern":dbl[], dbl[]})  [unwired: 1 in]
            n241 = Divide(x=w217, y=2.0) -> (x/y=w215:dbl)
            n242 = Threshold 1D Array(2:w215, 3:w207) -> (0:w211:dbl)  [unwired: 1 in]
            n243 = Compound Arithmetic op=ADD(w143, w144) -> (w142:dbl)
            n244 = Greater?(x=w202, y=1.0) -> (0:w249:bool)
            n245 = Index Array(array=w154, index=w209) -> (element=w208:dbl)
            n246 = Index Array(array=w154, index=w211) -> (element=w210:dbl)
            n247 = Absolute Value(x=w151) -> (abs(x)=w283:dbl)
            n248 = Subtract(x=w208, y=w210) -> (x-y=w214:dbl)
            n249 = Select(t=1.0 ("y"), s=w249, f=w202) -> (s? t:f=w201:dbl)
            n250 = Absolute Value(x=w214) -> (abs(x)=w213:dbl)
            n251 = Multiply(x=w213, y=2.0) -> (x*y=→"FWHM (eV)":dbl)
          }
          "e_FMO (y)" <- w106
        }
        "angle\narray\nfor sigma" <- w31
        "Array 2" <- w2
        "Array 3" <- w3
        n252 = Delete From Array(array=w5, index (col)=0 ("disabled index (col)")) -> ()  [unwired: 2 in, 2 out]
        n253 = Logarithm Base 10(1:w5) -> (0:w13:dbl[][])
        "log(G/G0) matrix" <- w13
        n254 = local read "e_FMO (y)"() -> (w20:dbl[])
        n255 = local read "angle\narray\nfor sigma"() -> (w4:dbl[])
        n256 = call-poly <vilib>:"Plot Helper.vi"("z matrix"=w13, "y vector"=w20, "x vector"=w4) -> ("3D Plot lvclass Array out"=→"log(G/G0)=f(angle, e_iso) for t(d-head)":refnum<class "3D Plot Datatype.lvclass">[])  [unwired: 3 in, 5 out]
        n257 = call-poly <vilib>:"Plot Helper.vi"("z matrix"=w11, "y vector"=w20, "x vector"=w4) -> ("3D Plot lvclass Array out"=→"Gamma(angle, e_iso) for t(d-head)_sum dz2 & dyz":refnum<class "3D Plot Datatype.lvclass">[])  [unwired: 3 in, 5 out]
        n258 = call-poly <vilib>:"Plot Helper.vi"("z matrix"=w12, "y vector"=w20, "x vector"=w4) -> ("3D Plot lvclass Array out"=→"Gamma(angle, e_iso) for t(sp-head)_sum pz & py":refnum<class "3D Plot Datatype.lvclass">[])  [unwired: 3 in, 5 out]
        n259 = call-poly <vilib>:"Plot Helper.vi"("z matrix"=w10, "y vector"=w20, "x vector"=w4) -> ("3D Plot lvclass Array out"=→"final ELA(angle, e_iso)  for t(d-head)":refnum<class "3D Plot Datatype.lvclass">[])  [unwired: 3 in, 5 out]
        n260 = call-poly <vilib>:"Plot Helper.vi"("z matrix"=w8, "y vector"=w20, "x vector"=w4) -> ("3D Plot lvclass Array out"=→"delta(angle, e_iso) for t(d-head)_sum dz2 & dyz":refnum<class "3D Plot Datatype.lvclass">[])  [unwired: 3 in, 5 out]
        n261 = call-poly <vilib>:"Plot Helper.vi"("z matrix"=w13, "y vector"=w20, "x vector"=w4) -> ("3D Plot lvclass Array out"=→"log(G/G0)=f(angle, e_iso) for t(sp-head)":refnum<class "3D Plot Datatype.lvclass">[])  [unwired: 3 in, 5 out]
        n262 = call-poly <vilib>:"Plot Helper.vi"("z matrix"=w9, "y vector"=w20, "x vector"=w4) -> ("3D Plot lvclass Array out"=→"delta(angle, e_iso) for t(sp-head)_only pz":refnum<class "3D Plot Datatype.lvclass">[])  [unwired: 3 in, 5 out]
        n263 = call-poly <vilib>:"Plot Helper.vi"("z matrix"=w10, "y vector"=w20, "x vector"=w4) -> ("3D Plot lvclass Array out"=→"final ELA(angle, e_iso  for t(sp-head))":refnum<class "3D Plot Datatype.lvclass">[])  [unwired: 3 in, 5 out]
        n264 = case shown="True" "save heatmap \n(sp band)?" {
          tunnel: w13 -> [_ w84]
          tunnel: w18 -> [_ w77]
          tunnel: w17 -> [_ w76]
          tunnel: "_delta shift=f(t, e_iso)" ("string") -> [_ w75]
          tunnel: w14 -> [_ w74]
          tunnel: w12 -> [_ w73]
          tunnel: w10 -> [_ w72]
          tunnel: w9 -> [_ w71]
          tunnel: w4 -> [_ w66]
          frame False {
          }
          frame True {
            w64 = ".txt"
            w63 = "_t(sp band-anchor) " ("string")
            w69 = TRUE ("transpose? (no:F)")
            w70 = "%#.10f" ("format (%.3f)")
            n265 = Concatenate Strings("name (sp band)", w63, w64) -> (w62:string)
            n266 = Concatenate Strings("name (sp band)", w77, w63, w64) -> (w85:string)
            n267 = Concatenate Strings("name (sp band)", w76, w63, w64) -> (w83:string)
            n268 = Concatenate Strings("name (sp band)", w75, w63, w64) -> (w81:string)
            n269 = Concatenate Strings("name (sp band)", w74, w63, w64) -> (w79:string)
            n270 = Build Path(base path="saving path_heatmap (sp band)", name or relative path=w62) -> (appended path=w67:path)
            n271 = Build Path(base path="saving path_heatmap (sp band)", name or relative path=w85) -> (appended path=w68:path)
            n272 = Build Path(base path="saving path_heatmap (sp band)", name or relative path=w83) -> (appended path=w82:path)
            n273 = Build Path(base path="saving path_heatmap (sp band)", name or relative path=w81) -> (appended path=w80:path)
            n274 = Build Path(base path="saving path_heatmap (sp band)", name or relative path=w79) -> (appended path=w78:path)
            n275 = call-poly <vilib>:"Write Delimited Spreadsheet.vi"("file path (dialog if empty)"=w67, "format (%.3f)"=w70, "1D data"=w66, "transpose? (no:F)"=w69) -> ()  [unwired: 10 in, 2 out]
            n276 = call-poly <vilib>:"Write Delimited Spreadsheet.vi"("file path (dialog if empty)"=w68, "format (%.3f)"=w70, "2D data"=w84, "transpose? (no:F)"=w69) -> ()  [unwired: 10 in, 2 out]
            n277 = call-poly <vilib>:"Write Delimited Spreadsheet.vi"("file path (dialog if empty)"=w82, "format (%.3f)"=w70, "2D data"=w73, "transpose? (no:F)"=w69) -> ()  [unwired: 10 in, 2 out]
            n278 = call-poly <vilib>:"Write Delimited Spreadsheet.vi"("file path (dialog if empty)"=w80, "format (%.3f)"=w70, "2D data"=w71, "transpose? (no:F)"=w69) -> ()  [unwired: 10 in, 2 out]
            n279 = call-poly <vilib>:"Write Delimited Spreadsheet.vi"("file path (dialog if empty)"=w78, "format (%.3f)"=w70, "2D data"=w72, "transpose? (no:F)"=w69) -> ()  [unwired: 10 in, 2 out]
          }
        }
        n280 = case shown="True" "save heatmap \n(d band)?" {
          tunnel: w18 -> [_ w52]
          tunnel: w17 -> [_ w51]
          tunnel: "_delta shift=f(t, e_iso)" ("string") -> [_ w50]
          tunnel: w14 -> [_ w49]
          tunnel: w13 -> [_ w48]
          tunnel: w11 -> [_ w47]
          tunnel: w10 -> [_ w46]
          tunnel: w8 -> [_ w45]
          tunnel: w4 -> [_ w36]
          frame False {
          }
          frame True {
            w37 = "_t(d band-anchor) " ("string")
            w38 = ".txt"
            w42 = "%#.10f" ("format (%.3f)")
            w41 = TRUE ("transpose? (no:F)")
            n281 = Concatenate Strings("name (d band)", w37, w38) -> (w44:string)
            n282 = Concatenate Strings("name (d band)", w51, w37, w38) -> (w55:string)
            n283 = Concatenate Strings("name (d band)", w52, w37, w38) -> (w53:string)
            n284 = Concatenate Strings("name (d band)", w50, w37, w38) -> (w57:string)
            n285 = Concatenate Strings("name (d band)", w49, w37, w38) -> (w59:string)
            n286 = Build Path(base path="saving path_heatmap (d band)", name or relative path=w44) -> (appended path=w43:path)
            n287 = Build Path(base path="saving path_heatmap (d band)", name or relative path=w55) -> (appended path=w56:path)
            n288 = Build Path(base path="saving path_heatmap (d band)", name or relative path=w53) -> (appended path=w54:path)
            n289 = Build Path(base path="saving path_heatmap (d band)", name or relative path=w57) -> (appended path=w58:path)
            n290 = Build Path(base path="saving path_heatmap (d band)", name or relative path=w59) -> (appended path=w60:path)
            n291 = call-poly <vilib>:"Write Delimited Spreadsheet.vi"("file path (dialog if empty)"=w43, "format (%.3f)"=w42, "1D data"=w36, "transpose? (no:F)"=w41) -> ()  [unwired: 10 in, 2 out]
            n292 = call-poly <vilib>:"Write Delimited Spreadsheet.vi"("file path (dialog if empty)"=w56, "format (%.3f)"=w42, "2D data"=w47, "transpose? (no:F)"=w41) -> ()  [unwired: 10 in, 2 out]
            n293 = call-poly <vilib>:"Write Delimited Spreadsheet.vi"("file path (dialog if empty)"=w54, "2D data"=w48, "transpose? (no:F)"=w41) -> ()  [unwired: 11 in, 2 out]
            n294 = call-poly <vilib>:"Write Delimited Spreadsheet.vi"("file path (dialog if empty)"=w58, "format (%.3f)"=w42, "2D data"=w45, "transpose? (no:F)"=w41) -> ()  [unwired: 10 in, 2 out]
            n295 = call-poly <vilib>:"Write Delimited Spreadsheet.vi"("file path (dialog if empty)"=w60, "format (%.3f)"=w42, "2D data"=w46, "transpose? (no:F)"=w41) -> ()  [unwired: 10 in, 2 out]
          }
        }
      }
      event Timeout {
        n296 = event-data() -> ()  [unwired: 1 in, 3 out]
      }
    }
  }
